vi "Plugin Page.vi"(8 "error in (no error)":errorcluster, 11 "Node Ptr":T2 format="%.0x") -> (0 "error out":errorcluster)   [LabVIEW 2017, in "DSF System Explorer.lvlib"]
uses:
  DSF System Explorer.lvlib
  <vilib>/NI Veristand/Custom Device API/Custom Device Item Ref.ctl
  DSF Core.lvlibp/Typedefs/DSF Configuration ID.ctl
  DSF Core.lvlibp/Classes/User Interface/Core/Plugin/Core Plugin User Interface.lvclass
  Get Settings ID (Plugin).vi
  <vilib>/NI Veristand/Custom Device API/Custom Device API.lvlib
  DSF Core.lvlibp/Classes/User Interface Handler/User Interface Handler.lvclass
  DSF Core.lvlibp/Classes/User Interface/Plugin/Component Settings Editor.lvclass
  DSF Core.lvlibp/Classes/Configuration Session/Configuration Session.lvclass
  C:/Git/DSF/VeriStand/Data Sharing Custom Device/Source/DSF Core.lvlibp/Classes/User Interface/User Interface.lvclass
  DSF Core.lvlibp
panel:
  out "settings id":T1={"plugin"=-1, "thread"=-1, "group"=-1, "transfer"=-1, "channel"=-1}
  in  "Header":cluster{"Section Name":string}={"Section Name"="Plugin"}
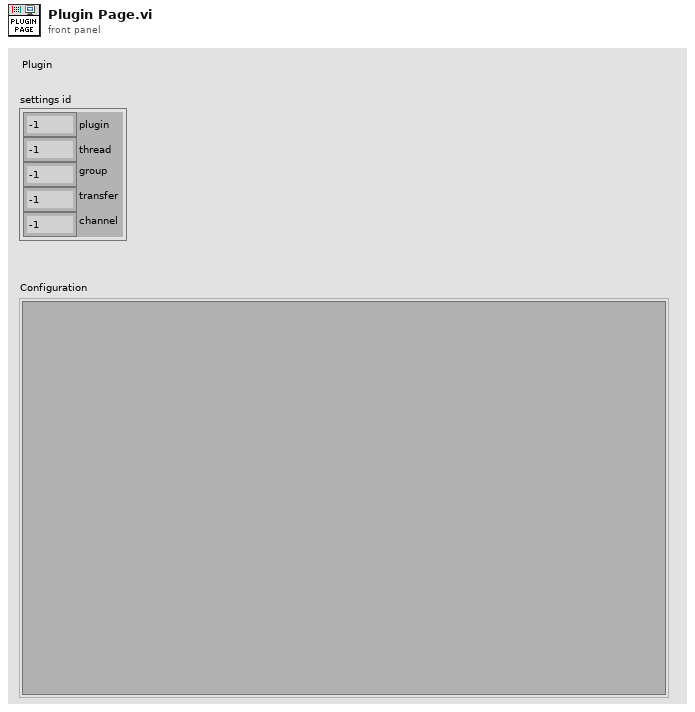
[diagram p1: front panel]
types:
  T1 = typedef "DSF Core.lvlibp/DSF Configuration ID.ctl" = cluster{"plugin":i32, "thread":i32, "group":i32, "transfer":i32, "channel":i32}
  T2 = typedef "Custom Device API.lvlib/Custom Device Item Ref.ctl" = u64
  T3 = typedef "Custom Device API.lvlib/Custom Device Commands.ctl" = enum16{"Default", "Item renamed", "Shutdown", "Dynamic button pressed"}
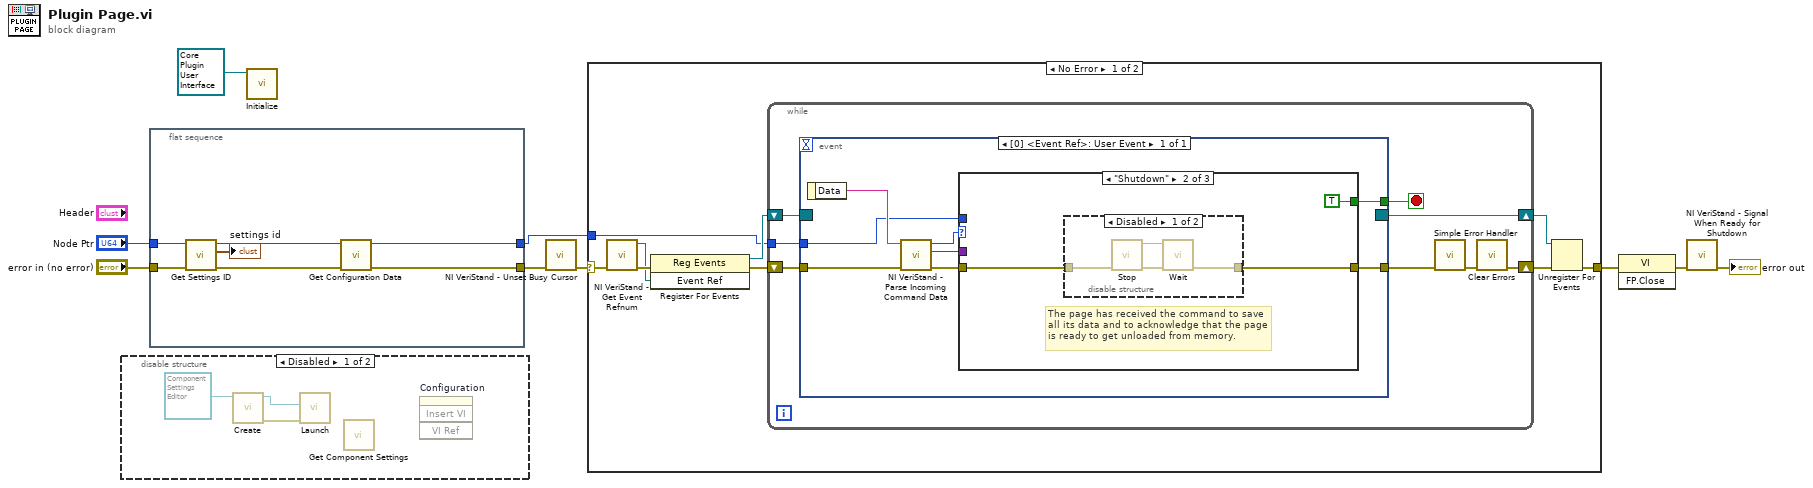
[diagram p0: block diagram]
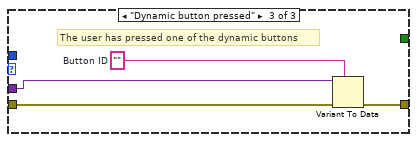
[diagram p5: hidden frame]
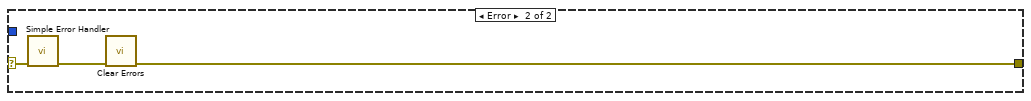
[diagram p6: hidden frame]
diagram:
  n1 = disable-structure shown="Disabled" {
    frame Disabled {
      n2 = call "Create.vi"("Component Settings Editor in"=refnum<class "Component Settings Editor.lvclass"> refnum ("DSF Core.lvlibp:Component Settings Editor.lvclass")) -> ("error out"=w11:errorcluster, "Component Settings Editor out"=w10:refnum<class "Component Settings Editor.lvclass">)  [unwired: 9 in]
      n3 = call "Launch.vi"("error in (no error)"=w11, "User Interface"=w10) -> ()  [unwired: 7 in, 3 out]
      n4 = call "Get Component Settings.vi"() -> ()  [unwired: 9 in, 3 out]
      n5 = invoke on="Configuration" class="SubPnl" method="Insert VI"() -> ()  [unwired: 4 in, 4 out]
    }
    frame Enabled {
    }
  }
  n6 = flat-sequence "Initialization code" {
    tunnel: "error in (no error)" -> [w19]
    tunnel: "Node Ptr" -> [w18]
    tunnel: [w14] -> w5
    tunnel: [w13] -> w2
    frame #0 {
      n7 = call-poly "Get Settings ID.vi"("error in (no error)"=w19, "Item Ref in"=w18) -> ("error out"=w16:errorcluster, "settings id"=→"settings id":T1, "Item Ref out"=w15:T2)  [unwired: 7 in]
      n8 = call "Get Configuration Data.vi"("error in (no error)"=w16, "Item Ref in"=w15) -> ("error out"=w14:errorcluster, "Item Ref out"=w13:T2)  [unwired: 7 in, 1 out]
    }
  }
  n9 = call-dynamic "Initialize.vi"("Core Plugin User Interface in"=refnum<class "Core Plugin User Interface.lvclass"> refnum ("DSF Core.lvlibp:Core Plugin User Interface.lvclass")) -> ()  [unwired: 9 in, 2 out]
  n10 = call <vilib>:"NI VeriStand - Unset Busy Cursor.vi"("error in (no error)"=w5) -> ("error out"=w4:errorcluster)  [unwired: 10 out]
  n11 = case shown="No Error" w4 {
    selector: w4 -> [w20 w60]
    tunnel: [w25 w58] -> w9
    tunnel: w2 -> [w21 _]
    frame No Error {
      n12 = call <vilib>:"NI VeriStand - Get Event Refnum.vi"("error in (no error)"=w20) -> ("error out"=w28:errorcluster, "Event Ref"=w24:refnum<user-event>)  [unwired: 9 out]
      n13 = register-events(error in=w28, w24) -> (reference out=w22:refnum<event-registration>, error out=w23:errorcluster)  [unwired: 1 in]
      n14 = while {
        tunnel: w21 -> [w32]
        shift-right: [w29] -> w26
        shift-left: w23 -> [w35]
        shift-right: [w36] -> w27
        shift-left: w22 -> [w34]
        stop <- w33 stop-if-true
        n15 = event shown="[0] <Event Ref>: User Event" {
          selector: w34 -> [_]
          dyn-events: [_] -> w36
          timeout: _ -> [_]
          tunnel: w35 -> [w44]
          tunnel: [w40] -> w33
          tunnel: [w39] -> w31
          tunnel: w32 -> [w38]
          event User Event {
            n16 = event-data() -> ("Data"=w43:string)  [unwired: 1 out]
            n17 = call <vilib>:"NI VeriStand - Parse Incoming Command Data.vi"("error in (no error)"=w44, "Incoming data"=w43) -> ("error out"=w42:errorcluster, "Outgoing data"=w37:variant, "Action"=w41:T3)  [unwired: 7 out]
            n18 = case shown="\"Shutdown\"" w41 {
              tunnel: w42 -> [w45 w47 w57]
              tunnel: [_ TRUE _] -> w40
              tunnel: [w45 w46 w54] -> w39
              tunnel: w38 -> [_ _ _]
              tunnel: w37 -> [_ _ w56]
              frame "Default", Default {
              }
              frame "Shutdown" {
                # "The page has received the command to save all its data and to acknowledge that the page is ready to get unloaded from memory."
                n19 = disable-structure shown="Disabled" {
                  disable-tunnel: w47 -> [w52 w53]
                  disable-tunnel: [w49 w53] -> w46
                  frame Disabled {
                    n20 = call "Stop.vi"("error in (no error)"=w52) -> ("error out"=w51:errorcluster, "User Interface Handler out"=w50:refnum<class "User Interface Handler.lvclass">)  [unwired: 9 in]
                    n21 = call "Wait.vi"("error in (no error)"=w51, "User Interface Handler in"=w50) -> ("error out"=w49:errorcluster)  [unwired: 7 in, 2 out]
                  }
                  frame Enabled {
                  }
                }
              }
              frame "Dynamic button pressed" {
                w55 = ""  # Button ID
                # "The user has pressed one of the dynamic buttons"
                n22 = Variant To Data(error in=w57, type=w55, Variant=w56) -> (error out=w54:errorcluster)  [unwired: 1 out]
              }
            }
          }
        }
        n23 = call <vilib>:"Simple Error Handler.vi"("error in (no error)"=w31) -> ("error out"=w30:errorcluster)  [unwired: 1 in, 7 out]
        n24 = call <vilib>:"Clear Errors.vi"("error in (no error)"=w30) -> ("error out"=w29:errorcluster)  [unwired: 1 in, 5 out]
      }
      n25 = Unregister For Events(event registration refnum=w27, error in=w26) -> (error out=w25:errorcluster)
    }
    frame Error {
      n26 = call <vilib>:"Simple Error Handler.vi"("error in (no error)"=w60) -> ("error out"=w59:errorcluster)  [unwired: 1 in, 7 out]
      n27 = call <vilib>:"Clear Errors.vi"("error in (no error)"=w59) -> ("error out"=w58:errorcluster)  [unwired: 1 in, 5 out]
    }
  }
  n28 = invoke class="VI" method="FP.Close"(error in=w9) -> (error out=w8:errorcluster)  [unwired: 2 in, 2 out]
  n29 = call <vilib>:"NI VeriStand - Signal When Ready for Shutdown.vi"("error in (no error)"=w8) -> ("error out"=→"error out":errorcluster)  [unwired: 10 out]
